vi "Format Entry.vi"(8 "error in (no error)":errorcluster, 10 "Log Data":T1={"Time"=timestamp(0 s since 1904-01-01), "Level"=enum."INFO", "Logger"="", "Message"="", "Arguments"=[]} {"Time" format="%<%x %.3X>T"}, 11 "CSVLayout in":refnum<class "CSVLayout.lvclass">) -> (0 "error out":errorcluster, 2 "Log Entry":string, 3 "CSVLayout out":refnum<class "CSVLayout.lvclass">)   [LabVIEW 2019, in "TSC Event Logger.lvlib" / "CSVLayout.lvclass"]
uses:
  CSVLayout.lvclass
  Log Data.ctl
  Log/Event Level.ctl
  Layout.lvclass
  TSC Event Logger.lvlib
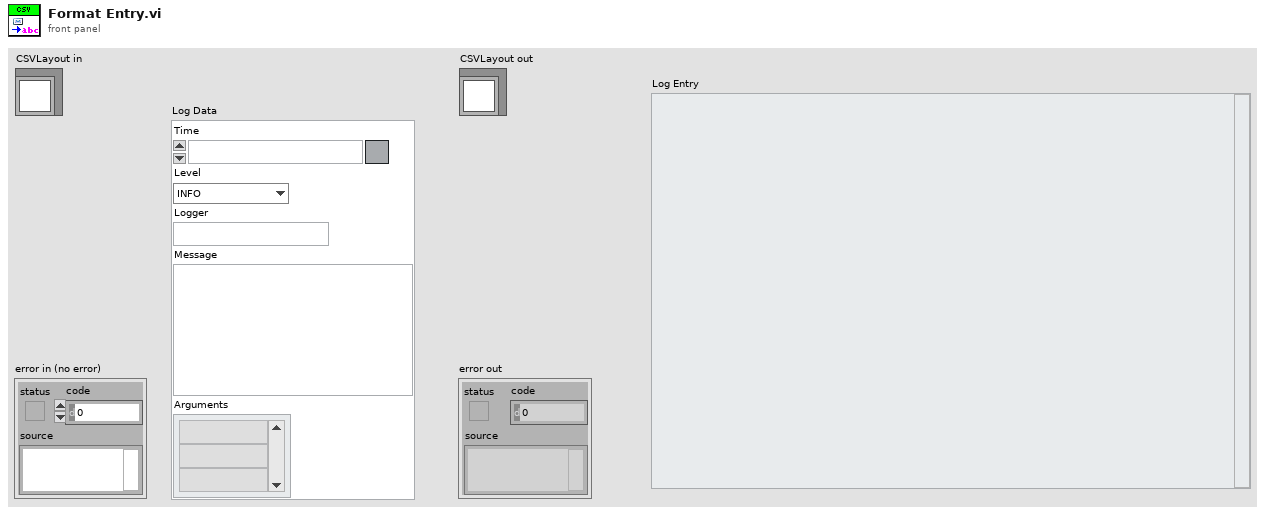
[diagram p1: front panel]
types:
  T1 = typedef "TSC Event Logger.lvlib/Log Data.ctl" = cluster{"Time":timestamp, "Level":T2, "Logger":string, "Message":string, "Arguments":string[]}
  T2 = typedef "TSC Event Logger.lvlib/Event Level.ctl" = enum16{"OFF", "TRACE", "DEBUG", "INFO", "WARN", "ERROR", "FATAL"}
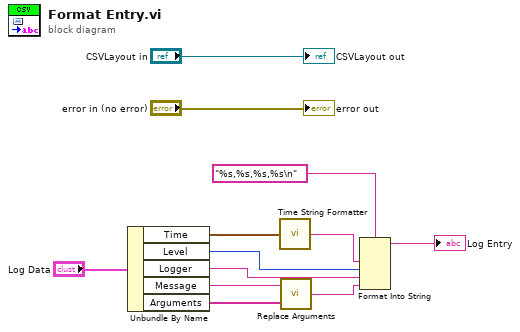
[diagram p0: block diagram]
diagram:
  n1 = Unbundle By Name("Log Data") -> ("Time"=w7:timestamp, "Level"=w9:T2, "Logger"=w8:string, "Message"=w5:string, "Arguments"=w4:string[])
  n2 = call "Time String Formatter.vi"("Time"=w7) -> ("Time string"=w6:string)
  n3 = call "Replace Arguments.vi"("Arguments"=w4, "Message"=w5) -> ("Output Message"=w3:string)
  n4 = Format Into String(format string="%s,%s,%s,%s\n", w6, w9, w8, w3) -> (resulting string=→"Log Entry":string)  [unwired: 2 in, 1 out]
  "error out" <- "error in (no error)"
  "CSVLayout out" <- "CSVLayout in"
